vi "tcsOfc_flushSamplesEvent_appliedSettingsMatchStart.vi"(8 "error in (no error)":errorcluster) -> (0 "error out":errorcluster, 3 "function return":i32)   [LabVIEW 2016, in "SALLV_tcsOfc.lvlib"]
doc: "int tcsOfc_shm_flushSamplesEvent_appliedSettingsMatchStartLV();"
uses:
  SALLV_tcsOfc.lvlib
  SALLV_tcsOfc.so
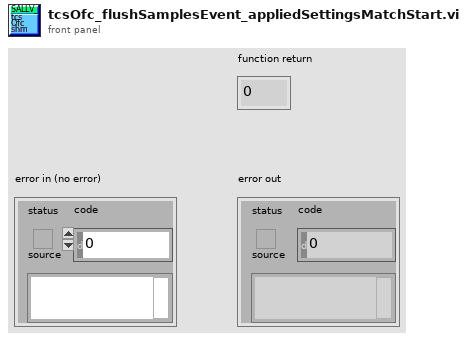
[diagram p1: front panel]
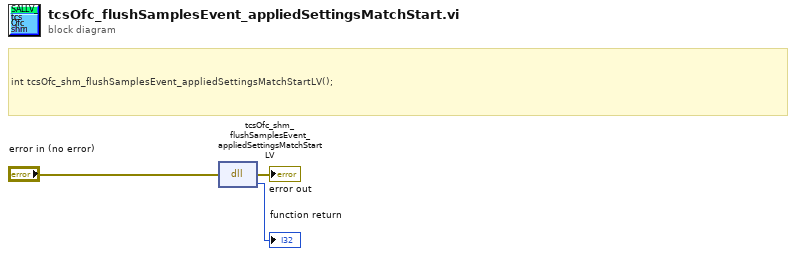
[diagram p0: block diagram]
diagram:
  # "int tcsOfc_shm_flushSamplesEvent_appliedSettingsMatchStartLV();"
  n1 = dll-call lib="home/ttsai/Documents/salAPI/SALLV_tcsOfc/SALLV_tcsOfc.*" fn="tcsOfc_shm_flushSamplesEvent_appliedSettingsMatchStartLV"(error in="error in (no error)") -> (error out=→"error out":errorcluster, →"function return":i32)  [unwired: 2 in, 1 out]
